vi "JsonFile_GetAttribute(Boolean).vi"(8 "error in (no error)":errorcluster, 9 "Default Value":bool, 10 "Attribute":string, 11 "Json":path) -> (0 "error out":errorcluster, 1 "Found?":bool, 2 "Value":bool, 3 "Json":path)   [LabVIEW 2019, in "lv-apt-json-file.lvlib"]
uses:
  <userlib>/_lvAPT/lv-apt-json-file/lv-apt-json-file.lvlib
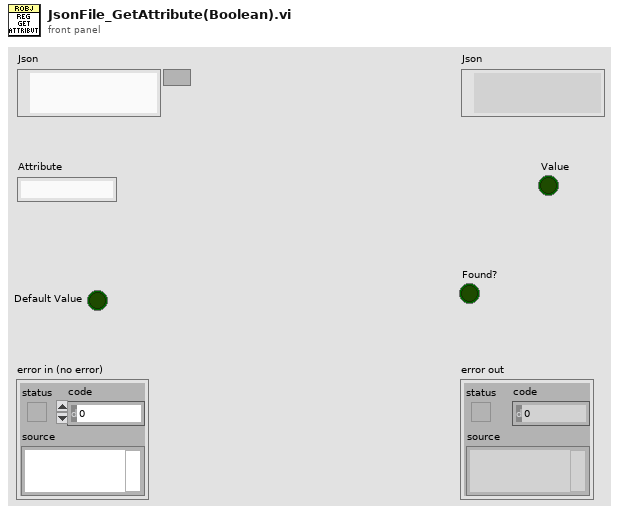
[diagram p1: front panel]
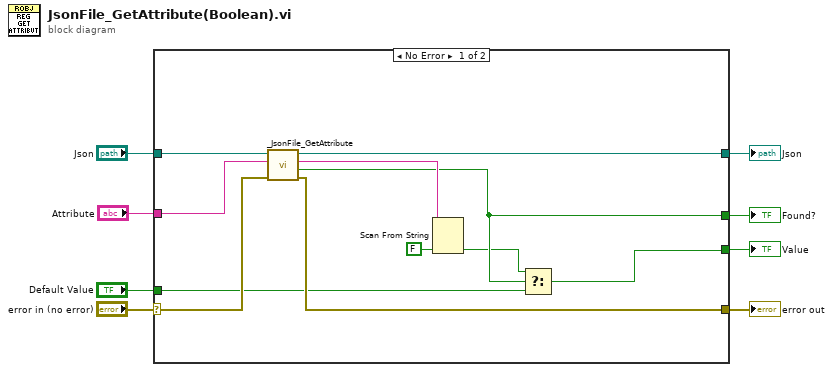
[diagram p0: block diagram]
diagram:
  n1 = case shown="No Error" "error in (no error)" {
    selector: "error in (no error)" -> [w17 w21]
    tunnel: "Json" -> [w18 w20]
    tunnel: "Attribute" -> [w19 _]
    tunnel: [w16 w20] -> w6
    tunnel: [w13 w21] -> w4
    tunnel: [w12 _] -> w3
    tunnel: [w9 _] -> w2
    tunnel: "Default Value" -> [w11 _]
    frame No Error {
      n2 = call <userlib>:"_JsonFile_GetAttribute.vi"("error in (no error)"=w17, "Attribute"=w19, "Json"=w18) -> ("error out"=w13:errorcluster, "Found?"=w12:bool, "String"=w15:string, "Json (dup)"=w16:path)  [unwired: 5 in]
      n3 = Scan From String(input string=w15, default 1=FALSE) -> (output 1=w10:bool)  [unwired: 3 in, 3 out]
      n4 = Select(t=w10, s=w12, f=w11) -> (s? t:f=w9:bool)
    }
    frame Error {
    }
  }
  "error out" <- w4
  "Json" <- w6
  "Value" <- w2
  "Found?" <- w3
